vi "Get URI.vi"(8 "error in (no error)":errorcluster, 11 "Endpoint in":refnum<class "Endpoint.lvclass">) -> (0 "error out":errorcluster, 2 "URI":refnum<class "URI.lvclass">, 3 "Endpoint out":refnum<class "Endpoint.lvclass">)   [LabVIEW 2020, in "Stream-Simple-Msg.lvlib" / "Endpoint.lvclass"]
doc: "Retrieves the URI of the endpoint connection. This typically shows the IP or hostname of the remote connection as well as any special parameters related to the connection."
uses:
  Endpoint.lvclass
  lv-stream/stream/URI/URI.lvclass
  Endpoint.lvclass/Endpoint.ctl
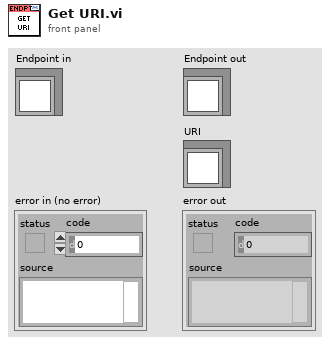
[diagram p1: front panel]
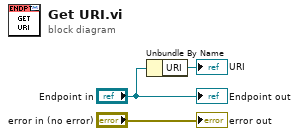
[diagram p0: block diagram]
diagram:
  n1 = Unbundle By Name("Endpoint in") -> ("URI"=→"URI":refnum<class "URI.lvclass">)
  "error out" <- "error in (no error)"
  "Endpoint out" <- "Endpoint in"
